vi "TestColision.vi"() -> ()   [LabVIEW 2017]
uses:
  Display/Display_mods.ctl
  Spaceship/Spaceship_mods.ctl
  ManageMovableObjects/ManRef_mods.ctl
  Asteroid/Asteroid_data.ctl
  GameConfig/GameConfig_data.ctl
  <vilib>/Utility/inputDevices.llb/keyboardAcquire.vi
  <userlib>/_OpenG.lib/numeric/numeric.llb/Random Number Within Range - DBL__ogtk.vi
  <userlib>/_OpenG.lib/numeric/numeric.llb/Random Number Within Range - I32__ogtk.vi
  <vilib>/Utility/inputDevices.llb/closeKeyboard.vi
panel:
  in  "Add":bool
  out "error out":errorcluster
  in  "stop":bool
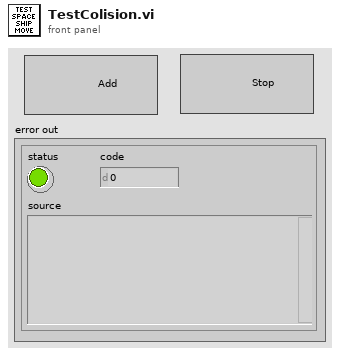
[diagram p1: front panel]
types:
  T1 = typedef "GameConfig_data.ctl" = cluster{"SpaceShip":cluster{"Angle":dbl, "SideLenght":dbl, "MaxLinearVeloc":dbl, "MaxAngularVeloc":dbl, "LinearAceleration":dbl, "AngularAceleration":dbl}, "Physics":cluster{"LinearDragFactor":dbl, "AngularDragFactor":dbl}, "Asteroids":cluster{"MaxSize":dbl, "MaxDivisions":i32, "MaxVeloc":dbl, "MinVeloc":dbl, "Fill":bool}, "Environment":cluster{"MaxAsteroids":i32, "TimeIncrement":dbl, "AsterProbCreation":dbl, "LogEnabled":bool}, "Shots":cluster{"MinTimeShots":dbl, "ShotSize":dbl, "ShotSpeed":dbl}}
  T2 = typedef "Display_mods.ctl" = enum16{"Init", "GetBase", "AddAster", "UpdateShip", "AddShoot", "DrawAll", "Clear", "Close"}
  T3 = typedef "ManRef_mods.ctl" = enum16{"Init", "NewAster", "MoveAll", "DestroyAster", "NewShoot", "DestroyShot", "CheckColision", "End"}
  T4 = typedef "Spaceship_mods.ctl" = enum16{"Init", "Move", "Rotate", "Translate", "GetData", "End"}
  T5 = typedef "Asteroid_data.ctl" = cluster{"Veloc":dbl, "Direction":dbl, "Size":i32, "displayRef":refnum<vi>, "Max X":dbl, "Max Y":dbl, "Xpos":dbl, "Ypos":dbl, "ID":i32, "Config":T1}
  T6 = enum16{"0", "1", "2", "3", "4", "5", "6", "7", "8", "9", "A", "B", "C", "D", "E", "F", "G", "H", "I", "J", "K", "L", "M", "N", "O", "P", "Q", "R", "S", "T", "U", "V", "W", "X", "Y", "Z", "F1", "F2", "F3", "F4", "F5", "F6", "F7", "F8", "F9", "F10", "F11", "F12", "F13", "F14", "F15", "ADD", "BACK", "BACKSLASH", "CAPITAL", "COMMA", "DECIMAL", "DELETE", "DIVIDE", "DOWN", "END", "EQUALS", "ESCAPE", "GRAVE (`)", "HOME", "INSERT", "LBRACKET", "LCONTROL", "LEFT", "L ALT", "LSHIFT", "LWIN", "MINUS", "MULTIPLY", "NEXT", "NUMLOCK", "NUMPAD_0", "NUMPAD_1", "NUMPAD_2", "NUMPAD_3", "NUMPAD_4", "NUMPAD_5", "NUMPAD_6", "NUMPAD_7", "NUMPAD_8", "NUMPAD_9", "PAUSE", "PERIOD", "PRIOR (PG UP)", "RBRACKET", "RCONTROL", "RETURN", "RIGHT", "R ALT", "RSHIFT", "RWIN", "SCROLL", "SEMICOLON", "SLASH", "SPACE", "SUBTRACT", "TAB", "UP", "ENTER (num pad)", "' (quote)"}[]
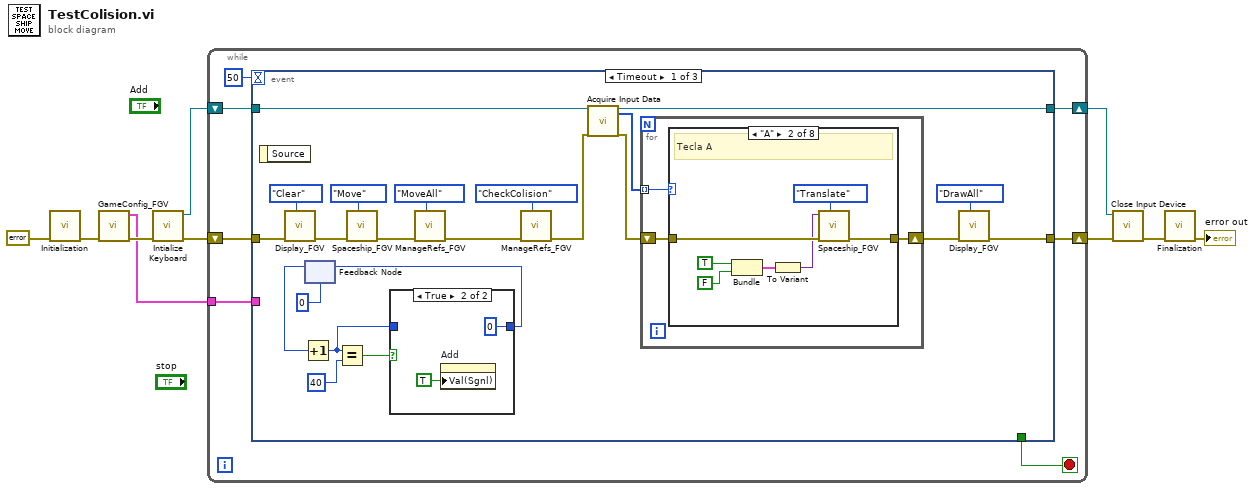
[diagram p0: block diagram]
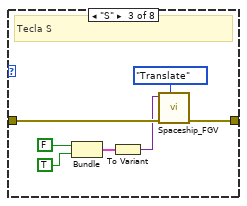
[diagram p4: hidden frame]
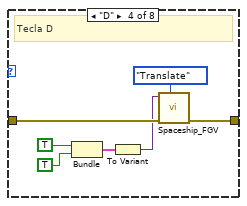
[diagram p5: hidden frame]
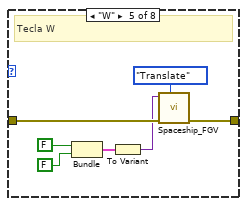
[diagram p6: hidden frame]
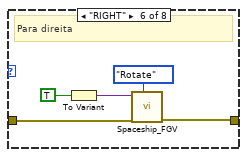
[diagram p7: hidden frame]
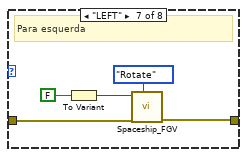
[diagram p8: hidden frame]
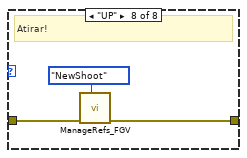
[diagram p9: hidden frame]
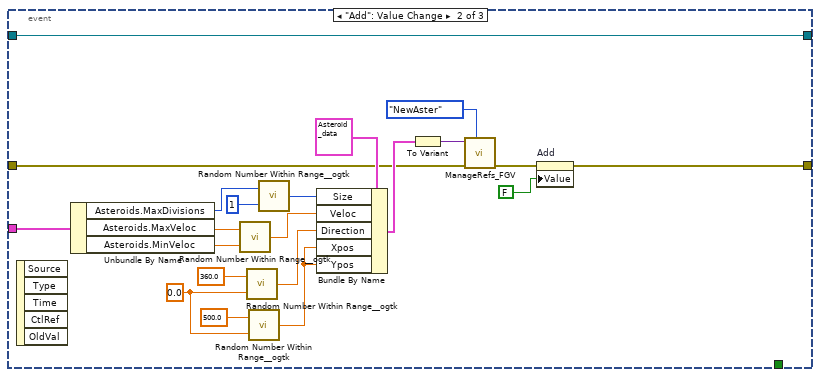
[diagram p10: hidden frame]
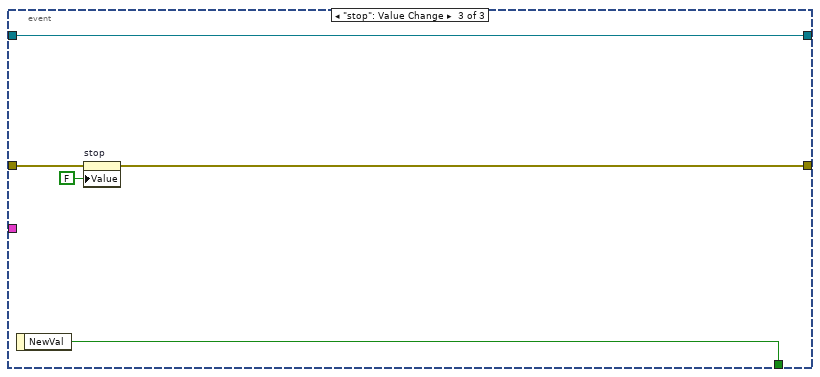
[diagram p11: hidden frame]
diagram:
  n1 = call "Initialization.vi"("error in"=errorcluster {"status"=FALSE, "code"=0, "source"=""}) -> ("error out"=w3:errorcluster)  [unwired: 10 in]
  n2 = call "GameConfig_FGV.vi"("error in"=w3) -> ("error out"=w2:errorcluster, "Config"=w1:T1)  [unwired: 9 in]
  n3 = call <vilib>:"Intialize Keyboard.vi"("error in (no error)"=w2) -> ("error out"=w8:errorcluster, "device ID"=w7:refnum<k1>)  [unwired: 9 in]
  n4 = while {
    shift-right: [w16] -> w6
    shift-left: w8 -> [w17]
    shift-right: [w12] -> w4
    shift-left: w7 -> [w13]
    tunnel: w1 -> [w11]
    stop <- w14 stop-if-true
    n5 = event shown="[0] Timeout" {
      selector: _ -> [_ _ _]
      dyn-events: _ -> [_ _ _]
      timeout: 50 -> [_ _ _]
      tunnel: w17 -> [w38 w92 w111]
      tunnel: [w18 w91 w110] -> w16
      tunnel: [_ _ w113] -> w14
      tunnel: w13 -> [w35 w88 w109]
      tunnel: [w34 w88 w109] -> w12
      tunnel: w11 -> [_ w89 _]
      event Timeout {
        n6 = event-data() -> ()  [unwired: 1 in, 1 out]
        n7 = call "Display_FGV.vi"("Display_mods"=Display_mods."Clear", "error in"=w38) -> ("error out"=w37:errorcluster)  [unwired: 8 in, 1 out]
        n8 = feedback #1(0) -> (w30:i32)
        n9 = Increment(x=w30) -> (x+1=w25:i32)
        n10 = Equal?(x=w25, y=40) -> (x = y?=w27:bool)
        n11 = call "Spaceship_FGV.vi"("Spaceship_mods"=Spaceship_mods."Move", "error in"=w37) -> ("error out"=w32:errorcluster)  [unwired: 8 in, 1 out]
        n12 = case shown="True" w27 {
          tunnel: [w40 0] -> w26
          tunnel: w25 -> [w40 _]
          frame False {
          }
          frame True {
            n13 = property on="Add" class="Bool (strict)"("Val(Sgnl)"=TRUE ("Value (Signaling)")) -> ()  [unwired: 2 in, 2 out]
          }
        }
        n14 = feedback-in #1(w26) -> ()
        n15 = call "ManageRefs_FGV.vi"("ManRef_mods"=ManRef_mods."MoveAll", "error in"=w32) -> ("error out"=w22:errorcluster)  [unwired: 8 in, 1 out]
        n16 = call "ManageRefs_FGV.vi"("ManRef_mods"=ManRef_mods."CheckColision", "error in"=w22) -> ("error out"=w23:errorcluster)  [unwired: 8 in, 1 out]
        n17 = call-poly <vilib>:"Acquire Input Data.vi"("device ID"=w35, "error in (no error)"=w23) -> ("device ID"=w34:refnum<k1>, "keys pressed"=w33:T6, "error out"=w21:errorcluster)  [unwired: 15 in]
        n18 = for {
          shift-right: [w44] -> w19
          shift-left: w21 -> [w45]
          tunnel: w33 -> [w43] mode=indexing
          n19 = case shown="\"A\"" w43 {
            tunnel: w45 -> [w46 w52 w59 w66 w73 w78 w83 w86]
            tunnel: [w46 w51 w58 w65 w72 w77 w82 w85] -> w44
            frame "0", Default {
            }
            frame "A" {
              # "Tecla A"
              n20 = Bundle("stop"=TRUE, "stop"=FALSE) -> (w50:cluster{"stop":bool, "stop":bool})  [unwired: 1 in]
              n21 = To Variant(anything=w50) -> (Variant=w49:variant)
              n22 = call "Spaceship_FGV.vi"("Spaceship_mods"=Spaceship_mods."Translate", "error in"=w52, "DataIn"=w49) -> ("error out"=w51:errorcluster)  [unwired: 7 in, 1 out]
            }
            frame "S" {
              # "Tecla S"
              n23 = Bundle("stop"=FALSE, "stop"=TRUE) -> (w57:cluster{"stop":bool, "stop":bool})  [unwired: 1 in]
              n24 = To Variant(anything=w57) -> (Variant=w56:variant)
              n25 = call "Spaceship_FGV.vi"("Spaceship_mods"=Spaceship_mods."Translate", "error in"=w59, "DataIn"=w56) -> ("error out"=w58:errorcluster)  [unwired: 7 in, 1 out]
            }
            frame "D" {
              # "Tecla D"
              n26 = Bundle("stop"=TRUE, "stop"=TRUE) -> (w64:cluster{"stop":bool, "stop":bool})  [unwired: 1 in]
              n27 = To Variant(anything=w64) -> (Variant=w63:variant)
              n28 = call "Spaceship_FGV.vi"("Spaceship_mods"=Spaceship_mods."Translate", "error in"=w66, "DataIn"=w63) -> ("error out"=w65:errorcluster)  [unwired: 7 in, 1 out]
            }
            frame "W" {
              # "Tecla W"
              n29 = Bundle("stop"=FALSE, "stop"=FALSE) -> (w71:cluster{"stop":bool, "stop":bool})  [unwired: 1 in]
              n30 = To Variant(anything=w71) -> (Variant=w70:variant)
              n31 = call "Spaceship_FGV.vi"("Spaceship_mods"=Spaceship_mods."Translate", "error in"=w73, "DataIn"=w70) -> ("error out"=w72:errorcluster)  [unwired: 7 in, 1 out]
            }
            frame "RIGHT" {
              # "Para direita"
              n32 = To Variant(anything=TRUE ("stop")) -> (Variant=w76:variant)
              n33 = call "Spaceship_FGV.vi"("Spaceship_mods"=Spaceship_mods."Rotate", "error in"=w78, "DataIn"=w76) -> ("error out"=w77:errorcluster)  [unwired: 7 in, 1 out]
            }
            frame "LEFT" {
              # "Para esquerda"
              n34 = To Variant(anything=FALSE ("stop")) -> (Variant=w81:variant)
              n35 = call "Spaceship_FGV.vi"("Spaceship_mods"=Spaceship_mods."Rotate", "error in"=w83, "DataIn"=w81) -> ("error out"=w82:errorcluster)  [unwired: 7 in, 1 out]
            }
            frame "UP" {
              # "Atirar!"
              n36 = call "ManageRefs_FGV.vi"("ManRef_mods"=ManRef_mods."NewShoot", "error in"=w86) -> ("error out"=w85:errorcluster)  [unwired: 8 in, 1 out]
            }
          }
        }
        n37 = call "Display_FGV.vi"("Display_mods"=Display_mods."DrawAll", "error in"=w19) -> ("error out"=w18:errorcluster)  [unwired: 8 in, 1 out]
      }
      event "Add": Value Change {
        w98 = 0.0 ("Low")
        n38 = event-data() -> ()  [unwired: 1 in, 5 out]
        n39 = Unbundle By Name(w89) -> ("Asteroids.MaxDivisions"=w104:i32, "Asteroids.MaxVeloc"=w102:dbl, "Asteroids.MinVeloc"=w103:dbl)
        n40 = call-poly <userlib>:"Random Number Within Range__ogtk.vi"("High"=w102, "Low"=w103) -> ("Random Number"=w106:dbl)  [unwired: 3 in]
        n41 = call-poly <userlib>:"Random Number Within Range__ogtk.vi"("High"=360.0, "Low"=w98) -> ("Random Number"=w107:dbl)  [unwired: 3 in]
        n42 = call-poly <userlib>:"Random Number Within Range__ogtk.vi"("High"=500.0, "Low"=w98) -> ("Random Number"=w90:dbl)  [unwired: 3 in]
        n43 = call-poly <userlib>:"Random Number Within Range__ogtk.vi"("High"=w104, "Low"=1) -> ("Random Number"=w105:i32)  [unwired: 3 in]
        n44 = Bundle By Name(cluster=T5 {"Veloc"=100.0, "Direction"=0.0, "Size"=3, "displayRef"=refnum, "Max X"=0.0, "Max Y"=0.0, "Xpos"=0.0, "Ypos"=150.0, "ID"=0, "Config"={"SpaceShip"={"Angle"=30.0, "SideLenght"=2.0, "MaxLinearVeloc"=10.0, "MaxAngularVeloc"=10.0, "LinearAceleration"=1.0, "AngularAceleration"=1.0}, "Physics"={"LinearDragFactor"=1.0, "AngularDragFactor"=1.0}, "Asteroids"={"MaxSize"=6.0, "MaxDivisions"=3, "MaxVeloc"=8.0, "MinVeloc"=1.0, "Fill"=FALSE}, "Environment"={"MaxAsteroids"=10, "TimeIncrement"=0.1, "AsterProbCreation"=0.1, "LogEnabled"=FALSE}, "Shots"={"MinTimeShots"=10.0, "ShotSize"=0.1, "ShotSpeed"=0.1}}} ("AsteroidData"), "Size"=w105, "Veloc"=w106, "Direction"=w107, "Xpos"=w90, "Ypos"=w90) -> (w108:T5)
        n45 = To Variant(anything=w108) -> (Variant=w100:variant)
        n46 = call "ManageRefs_FGV.vi"("ManRef_mods"=ManRef_mods."NewAster", "error in"=w92, "DataIn"=w100) -> ("error out"=w101:errorcluster)  [unwired: 7 in, 1 out]
        n47 = property on="Add" class="Bool (strict)"(error in=w101, "Value"=FALSE ("Add")) -> (error out=w91:errorcluster)  [unwired: 1 in, 1 out]
      }
      event "stop": Value Change {
        n48 = event-data() -> ("NewVal"=w113:bool)  [unwired: 1 in]
        n49 = property on="stop" class="Bool (strict)"(error in=w111, "Value"=FALSE ("Add")) -> (error out=w110:errorcluster)  [unwired: 1 in, 1 out]
      }
    }
  }
  n50 = call-poly <vilib>:"Close Input Device.vi"("error in (no error)"=w6, "device ID"=w4) -> ("error out"=w5:errorcluster)  [unwired: 8 in]
  n51 = call "Finalization.vi"("error in"=w5) -> ("error out"=→"error out":errorcluster)  [unwired: 10 in]
